vi "FPGA-Start-05-17.vi"() -> (0 "error out":errorcluster, 1 "FPGA VI Reference Out":refnum<k20>)   [LabVIEW 2010]
uses:
  <vilib>/userDefined/High Color/nirio_resource_hc.ctl
  <vilib>/rvi/interface/nirviOpenFPGA/nirviOpenFPGA.xnode
  <vilib>/rvi/interface/nirviMethod/nirviMethod.xnode
  <vilib>/LabVIEW Targets/FPGA/cRIO/shared/nicrio_ModuleControls/nicrio_cRIO-9871_FlowControlEnum.ctl
  <vilib>/LabVIEW Targets/FPGA/cRIO/shared/nicrio_ModuleControls/nicrio_cRIO-9871_StopBitsEnum.ctl
  <vilib>/LabVIEW Targets/FPGA/cRIO/shared/nicrio_ModuleControls/nicrio_cRIO-9871_ParityEnum.ctl
  <vilib>/LabVIEW Targets/FPGA/cRIO/shared/nicrio_ModuleControls/nicrio_cRIO-9871_DataBitsEnum.ctl
  <vilib>/LabVIEW Targets/FPGA/cRIO/shared/nicrio_ModuleControls/nicrio_cRIO-9871_BaudRateEnum.ctl
  <vilib>/rvi/interface/nirviReadWriteControl/nirviReadWriteControl.xnode
  <vilib>/Utility/error.llb/Error Cluster From Error Code.vi
  <vilib>/rvi/errors/niLvFpgaWhatHappensToTopLevelVI.ctl
  <vilib>/rvi/interface/common/niFpgaNodeNameForErrorReporting.ctl
  <vilib>/rvi/errors/niLvFpgaAdjustHostInterfaceError.vi
  NiFpgaLv.dll
  C:/Users/HAGAR-IV/Desktop/Zeugs/Johnny/pertrasgc fpga/FPGA-Programm-05-17.vi
  <vilib>/FPGAPlugInAG/cRIO-9114/niLvFpga_Reset_cRIO-9114.vi
  C:/Users/HAGAR-IV/Desktop/Zeugs/markus/version feb 2012/FPGA Bitfiles/pertrasgcfpga2_FPGATarget_FPGA-Programm-05_A75D3647.lvbitx
  <vilib>/FPGAPlugInAG/cRIO-9114/niLvFpga_Open_cRIO-9114.vi
  <vilib>/rvi/ClientSDK/nirviWhatTheDeviceIsDoing.ctl
  <vilib>/RVI Host/nirviSupport.llb/nirviErrorClusterFromErrorCode.vi
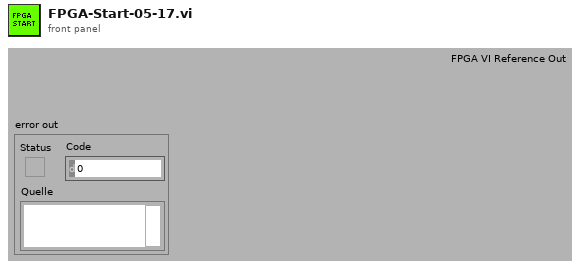
[diagram p1: front panel]
types:
  T1 = cluster{"H1-Valve2":u32, "H1-Spare2":u32, "H1-Spare1":u32, "H1-Valve1":u32, "H0-Drier":u32, "HL-Licor":u32, "H2-ECD2":u32, "H2-Oven":u32, "H2-Spare1":u32, "H2-Col2":u32, "H2-Col1":u32, "H2-ECD1":u32}
  T2 = cluster{"H1-Valve2":bool, "H1-Spare2":bool, "H1-Spare1":bool, "H1-Valve1":bool, "H0-Drier":bool, "HL-Licor":bool, "H2-ECD2":bool, "H2-Oven":bool, "H2-Spare1":bool, "H2-Col2":bool, "H2-Col1":bool, "H2-ECD1":bool}
  T3 = cluster{"Mod6/DIO 0":bool, "Mod6/DIO 1":bool, "Mod6/DIO 2":bool, "Mod6/DIO 3":bool, "Mod6/DIO 4":bool, "Mod6/DIO 5":bool, "Mod6/DIO 6":bool, "Mod6/DIO 7":bool, "Mod6/DIO 8":bool, "Mod6/DIO 9":bool, "Mod6/DIO 10":bool, "Mod6/DIO 11":bool, "Mod6/DIO 12":bool, "Mod6/DIO 13":bool, "Mod6/DIO 14":bool, "Mod6/DIO 15":bool, "Mod6/DIO 16":bool, "Mod6/DIO 17":bool, "Mod6/DIO 18":bool, "Mod6/DIO 19":bool, "Mod6/DIO 20":bool, "Mod6/DIO 21":bool, "Mod6/DIO 22":bool, "Mod6/DIO 23":bool, "Mod6/DIO 24":bool, "Mod6/DIO 25":bool, "Mod6/DIO 26":bool, "Mod6/DIO 27":bool, "Mod6/DIO 28":bool, "Mod6/DIO 29":bool, "Mod6/DIO 30":bool, "Mod6/DIO 31":bool}
  T4 = cluster{"Mod5/DIO 0":bool, "Mod5/DIO 1":bool, "Mod5/DIO 2":bool, "Mod5/DIO 3":bool, "Mod5/DIO 4":bool, "Mod5/DIO 5":bool, "Mod5/DIO 6":bool, "Mod5/DIO 7":bool, "Mod5/DIO 8":bool, "Mod5/DIO 9":bool, "Mod5/DIO 10":bool, "Mod5/DIO 11":bool, "Mod5/DIO 12":bool, "Mod5/DIO 13":bool, "Mod5/DIO 14":bool, "Mod5/DIO 15":bool, "Mod5/DIO 16":bool, "Mod5/DIO 17":bool, "Mod5/DIO 18":bool, "Mod5/DIO 19":bool, "Mod5/DIO 20":bool, "Mod5/DIO 21":bool, "Mod5/DIO 22":bool, "Mod5/DIO 23":bool, "Mod5/DIO 24":bool, "Mod5/DIO 25":bool, "Mod5/DIO 26":bool, "Mod5/DIO 27":bool, "Mod5/DIO 28":bool, "Mod5/DIO 29":bool, "Mod5/DIO 30":bool, "Mod5/DIO 31":bool}
  T5 = cluster{"proportional gain (Kc)":fxp<+/-,16,8>, "integral gain (Kc*Ts/Ti)":fxp<+/-,16,8>, "derivative gain (Kc*Td/Ts)":fxp<+/-,16,8>}
  T6 = typedef "nicrio_cRIO-9871_BaudRateEnum.ctl" = enum16{"75 bps", "110 bps", "134 bps", "150 bps", "300 bps", "600 bps", "1200 bps", "1800 bps", "2400 bps", "4800 bps", "7200 bps", "9600 bps", "14.4 kbps", "19.2 kbps", "28.8 kbps", "38.4 kbps", "57.6 kbps", "115.2 kbps", "230.4 kbps", "460.8 kbps", "921.6 kbps"}
  T7 = typedef "nicrio_cRIO-9871_DataBitsEnum.ctl" = enum8{"5", "6", "7", "8"}
  T8 = typedef "nicrio_cRIO-9871_ParityEnum.ctl" = enum8{"None", "Odd", "Even", "Mark", "Space"}
  T9 = typedef "nicrio_cRIO-9871_StopBitsEnum.ctl" = enum8{"1", "1.5", "2"}
  T10 = typedef "nicrio_cRIO-9871_FlowControlEnum.ctl" = enum8{"None", "Software (XON / XOFF)", "Hardware (RTS / CTS)"}
  T11 = cluster{"Mod7/Port1":cluster{"Baud Rate":T6, "Data Bits":T7, "Parity":T8, "Stop Bits":T9, "Flow Control":T10}, "Mod7/Port2":cluster{"Baud Rate":T6, "Data Bits":T7, "Parity":T8, "Stop Bits":T9, "Flow Control":T10}, "Mod7/Port3":cluster{"Baud Rate":T6, "Data Bits":T7, "Parity":T8, "Stop Bits":T9, "Flow Control":T10}, "Mod7/Port4":cluster{"Baud Rate":T6, "Data Bits":T7, "Parity":T8, "Stop Bits":T9, "Flow Control":T10}, "Mod8/Port1":cluster{"Baud Rate":T6, "Data Bits":T7, "Parity":T8, "Stop Bits":T9, "Flow Control":T10}, "Mod8/Port2":cluster{"Baud Rate":T6, "Data Bits":T7, "Parity":T8, "Stop Bits":T9, "Flow Control":T10}, "Mod8/Port3":cluster{"Baud Rate":T6, "Data Bits":T7, "Parity":T8, "Stop Bits":T9, "Flow Control":T10}, "Mod8/Port4":cluster{"Baud Rate":T6, "Data Bits":T7, "Parity":T8, "Stop Bits":T9, "Flow Control":T10}}
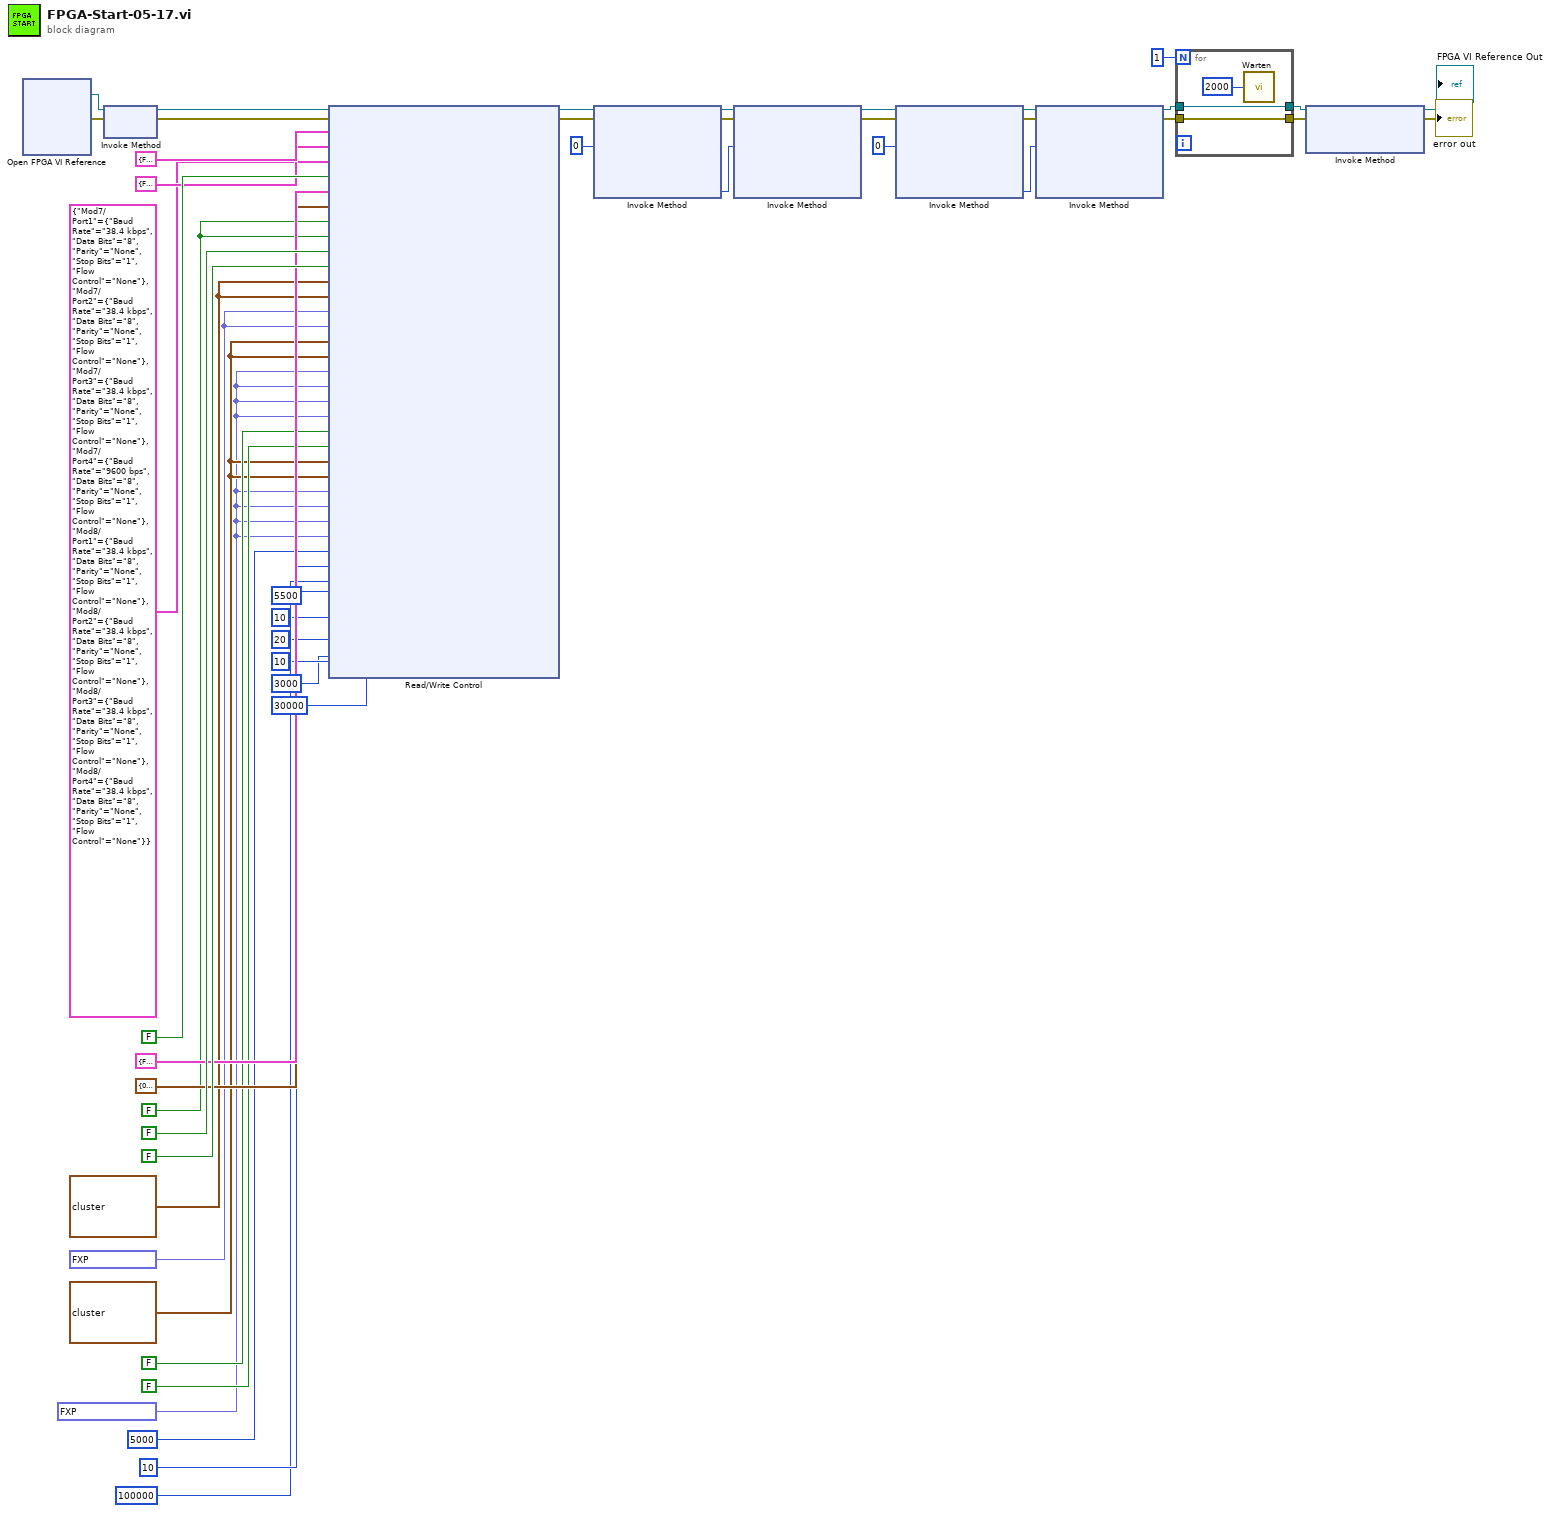
[diagram p0: block diagram]
diagram:
  w11 = fxp<+/-,16,6> 0.0 ("SetpointTrap1")
  w14 = fxp<+/-,16,4> 0.0 ("Umax[V]Mach1")
  w15 = T5 {"proportional gain (Kc)"=0.0, "integral gain (Kc*Ts/Ti)"=0.0, "derivative gain (Kc*Td/Ts)"=0.0} ("PIDMach1")
  w12 = T5 {"proportional gain (Kc)"=0.0, "integral gain (Kc*Ts/Ti)"=0.0, "derivative gain (Kc*Td/Ts)"=0.0} ("PIDTrap1")
  w13 = FALSE ("Heizen?Trap1")
  n1 = xnode "Open FPGA VI Reference"() -> ("FPGA VI Reference Out"=w22:refnum<k20>, "error out"=w21:errorcluster)  [unwired: 2 in]
  n2 = xnode "Invoke Method"("FPGA VI Reference In"=w22, "error in"=w21) -> ("FPGA VI Reference Out"=w42:refnum<k20>, "error out"=w43:errorcluster)
  n3 = xnode "Read/Write Control"("FPGA VI Reference In"=w42, "error in"=w43, "Mod5/DIO"=T4 {"Mod5/DIO 0"=FALSE, "Mod5/DIO 1"=FALSE, "Mod5/DIO 2"=FALSE, "Mod5/DIO 3"=FALSE, "Mod5/DIO 4"=FALSE, "Mod5/DIO 5"=FALSE, "Mod5/DIO 6"=FALSE, "Mod5/DIO 7"=FALSE, "Mod5/DIO 8"=FALSE, "Mod5/DIO 9"=FALSE, "Mod5/DIO 10"=FALSE, "Mod5/DIO 11"=FALSE, "Mod5/DIO 12"=FALSE, "Mod5/DIO 13"=FALSE, "Mod5/DIO 14"=FALSE, "Mod5/DIO 15"=FALSE, "Mod5/DIO 16"=FALSE, "Mod5/DIO 17"=FALSE, "Mod5/DIO 18"=FALSE, "Mod5/DIO 19"=FALSE, "Mod5/DIO 20"=FALSE, "Mod5/DIO 21"=FALSE, "Mod5/DIO 22"=FALSE, "Mod5/DIO 23"=FALSE, "Mod5/DIO 24"=FALSE, "Mod5/DIO 25"=FALSE, "Mod5/DIO 26"=FALSE, "Mod5/DIO 27"=FALSE, "Mod5/DIO 28"=FALSE, "Mod5/DIO 29"=FALSE, "Mod5/DIO 30"=FALSE, "Mod5/DIO 31"=FALSE}, "Mod6/DIO"=T3 {"Mod6/DIO 0"=FALSE, "Mod6/DIO 1"=FALSE, "Mod6/DIO 2"=FALSE, "Mod6/DIO 3"=FALSE, "Mod6/DIO 4"=FALSE, "Mod6/DIO 5"=FALSE, "Mod6/DIO 6"=FALSE, "Mod6/DIO 7"=FALSE, "Mod6/DIO 8"=FALSE, "Mod6/DIO 9"=FALSE, "Mod6/DIO 10"=FALSE, "Mod6/DIO 11"=FALSE, "Mod6/DIO 12"=FALSE, "Mod6/DIO 13"=FALSE, "Mod6/DIO 14"=FALSE, "Mod6/DIO 15"=FALSE, "Mod6/DIO 16"=FALSE, "Mod6/DIO 17"=FALSE, "Mod6/DIO 18"=FALSE, "Mod6/DIO 19"=FALSE, "Mod6/DIO 20"=FALSE, "Mod6/DIO 21"=FALSE, "Mod6/DIO 22"=FALSE, "Mod6/DIO 23"=FALSE, "Mod6/DIO 24"=FALSE, "Mod6/DIO 25"=FALSE, "Mod6/DIO 26"=FALSE, "Mod6/DIO 27"=FALSE, "Mod6/DIO 28"=FALSE, "Mod6/DIO 29"=FALSE, "Mod6/DIO 30"=FALSE, "Mod6/DIO 31"=FALSE}, "KonfigSeriell"=T11 {"Mod7/Port1"={"Baud Rate"=enum."38.4 kbps", "Data Bits"=enum."8", "Parity"=enum."None", "Stop Bits"=enum."1", "Flow Control"=enum."None"}, "Mod7/Port2"={"Baud Rate"=enum."38.4 kbps", "Data Bits"=enum."8", "Parity"=enum."None", "Stop Bits"=enum."1", "Flow Control"=enum."None"}, "Mod7/Port3"={"Baud Rate"=enum."38.4 kbps", "Data Bits"=enum."8", "Parity"=enum."None", "Stop Bits"=enum."1", "Flow Control"=enum."None"}, "Mod7/Port4"={"Baud Rate"=enum."9600 bps", "Data Bits"=enum."8", "Parity"=enum."None", "Stop Bits"=enum."1", "Flow Control"=enum."None"}, "Mod8/Port1"={"Baud Rate"=enum."38.4 kbps", "Data Bits"=enum."8", "Parity"=enum."None", "Stop Bits"=enum."1", "Flow Control"=enum."None"}, "Mod8/Port2"={"Baud Rate"=enum."38.4 kbps", "Data Bits"=enum."8", "Parity"=enum."None", "Stop Bits"=enum."1", "Flow Control"=enum."None"}, "Mod8/Port3"={"Baud Rate"=enum."38.4 kbps", "Data Bits"=enum."8", "Parity"=enum."None", "Stop Bits"=enum."1", "Flow Control"=enum."None"}, "Mod8/Port4"={"Baud Rate"=enum."38.4 kbps", "Data Bits"=enum."8", "Parity"=enum."None", "Stop Bits"=enum."1", "Flow Control"=enum."None"}}, "FIFO leer"=FALSE, "LHHeizen?"=T2 {"H1-Valve2"=FALSE, "H1-Spare2"=FALSE, "H1-Spare1"=FALSE, "H1-Valve1"=FALSE, "H0-Drier"=FALSE, "HL-Licor"=FALSE, "H2-ECD2"=FALSE, "H2-Oven"=FALSE, "H2-Spare1"=FALSE, "H2-Col2"=FALSE, "H2-Col1"=FALSE, "H2-ECD1"=FALSE}, "LHPulse(us)"=T1 {"H1-Valve2"=0, "H1-Spare2"=0, "H1-Spare1"=0, "H1-Valve1"=0, "H0-Drier"=0, "HL-Licor"=0, "H2-ECD2"=0, "H2-Oven"=0, "H2-Spare1"=0, "H2-Col2"=0, "H2-Col1"=0, "H2-ECD1"=0}, "Heizen?Trap1"=w13, "Heizen?Trap2"=w13, "Heizen?PreMach1"=FALSE ("Heizen?Mach1"), "Heizen?PreMach2"=FALSE ("Heizen?Mach2"), "PIDTrap1"=w12, "PIDTrap2"=w12, "SetpointTrap1"=w11, "SetpointTrap2"=w11, "PIDPreMach1"=w15, "PIDPreMach2"=w15, "Umax[V]PreMach1"=w14, "Umax[V]PreMach2"=w14, "USetp[V]PreMach1"=w14, "USetp[V]PreMach2"=w14, "Heizen?MainMach1"=FALSE, "Heizen?MainMach2"=FALSE, "PIDMainMach1"=w15, "PIDMainMach2"=w15, "Umax[V]MainMach1"=w14, "Umax[V]MainMach2"=w14, "USetp[V]MainMach1"=w14, "USetp[V]MainMach2"=w14, "Warten(us)"=u16 5000, "zwischenMesswerten(us)"=u16 10, "Periode(us)"=u32 100000, "5Van(us)"=u16 5500, "Messwerte"=10, "Abstand zwischen Messungen [us]Mach"=u16 20, "wie viele Messwerte?Mach"=u16 10, "vor der Messung [us]Mach"=u16 3000, "Per[us]Mach"=u16 30000) -> ("FPGA VI Reference Out"=w24:refnum<k20>, "error out"=w23:errorcluster)
  n4 = xnode "Invoke Method"("FPGA VI Reference In"=w24, "error in"=w23, "Number of Elements"=u32 0) -> ("FPGA VI Reference Out"=w47:refnum<k20>, "error out"=w44:errorcluster, "Elements Remaining"=w46:u32)  [unwired: 1 in, 1 out]
  n5 = xnode "Invoke Method"("FPGA VI Reference In"=w47, "error in"=w44, "Number of Elements"=w46) -> ("FPGA VI Reference Out"=w40:refnum<k20>, "error out"=w36:errorcluster)  [unwired: 1 in, 2 out]
  n6 = xnode "Invoke Method"("FPGA VI Reference In"=w40, "error in"=w36, "Number of Elements"=u32 0) -> ("FPGA VI Reference Out"=w38:refnum<k20>, "error out"=w35:errorcluster, "Elements Remaining"=w37:u32)  [unwired: 1 in, 1 out]
  n7 = xnode "Invoke Method"("FPGA VI Reference In"=w38, "error in"=w35, "Number of Elements"=w37) -> ("FPGA VI Reference Out"=w26:refnum<k20>, "error out"=w25:errorcluster)  [unwired: 1 in, 2 out]
  n8 = for {
    N: 1 -> [_]
    tunnel: w26 -> [w50]
    tunnel: [w50] -> w30
    tunnel: w25 -> [w49]
    tunnel: [w49] -> w28
    n9 = call "Warten"("Count(mSec)"=u32 2000) -> ()  [unwired: 1 out]
  }
  n10 = xnode "Invoke Method"("FPGA VI Reference In"=w30, "error in"=w28) -> ("FPGA VI Reference Out"=→"FPGA VI Reference Out":refnum<k20>, "error out"=→"error out":errorcluster)  [unwired: 1 in]
